vi "Main.vi"(11 "Module Admin":refnum<class "Delacor_lib_QMH_Module Admin.lvclass">) -> ()   [LabVIEW 2021, in "Signal Generator.lvlib"]
doc: "This template is based off of the Queued Message Handler design pattern and the Queued Message Handler project template that ships with LabVIEW.\n\nThe main difference is that the queue is private to this module and communication between modules is performed via Broadcast and Request events.\n\nRequest events are wrapped in public API methods and are handled in the Event Handling Loop (EHL) of this VI. Any module can register for Broadcast events sent by this module. The EHL generates messages based on user interface actions.\n\nThe Message Handling Loop (MHL) processes messages generated by the EHL, or by other messages. The messages are string values, so new messages can be added easily to the Message Cases case structure in the MHL. Each message cluster can also provide an optional value for Message Data, which is a variant that can be converted to whatever message-specific data is required.\n_____\nBased on DQMH Project Template 7.0.1.1316."
uses:
  Signal Generator.lvlib
  <vilib>/Delacor/Delacor QMH/Libraries/Module Admin_class/Delacor_lib_QMH_Module Admin.lvclass
  Module Data--cluster.ctl
  Update Parameters Argument--cluster.ctl
  <vilib>/Delacor/Delacor QMH/Libraries/Message Queue_class/Delacor_lib_QMH_Message Queue.lvclass/Delacor_lib_QMH_Message Queue.ctl
  Stop Argument--cluster.ctl
  <vilib>/Delacor/Delacor QMH/Libraries/Module Admin_class/Delacor_lib_QMH_Module Admin.lvclass/Delacor_lib_QMH_Module Admin.ctl
  Get Modules Name Argument--cluster.ctl
  Get Modules Name (Reply Payload)--cluster.ctl
  Update Parameters 2 Argument--cluster.ctl
  <vilib>/Utility/miscctls.llb/LVPointTypeDef.ctl
  <vilib>/Delacor/Delacor QMH/Libraries/Message Queue_class/Delacor_lib_QMH_Enqueue Message (Single).vi
  <vilib>/Delacor/Delacor QMH/Libraries/Module Admin_class/Delacor_lib_QMH_Get External Launch.vi
  <vilib>/Delacor/Delacor QMH/Libraries/Message Queue_class/Delacor_lib_QMH_Message Queue.lvclass
  <vilib>/measure/NI_MABase.lvlib
panel:
  out "error out":errorcluster
  out "Status":string
  in  "Simulate MHL Error":bool
  in  "Simulate EHL Error":bool
  # "Other processes communicate with this Module via its Public API (wrappers for its Request Events).\n\nThis Module communicates with other processes via its Broadcast Events.\nAny process that wants to receive these messages can register for this module's Broadcast events."
  # "This template is for the DQMH framework. See the block diagram for more information on how to use this template."
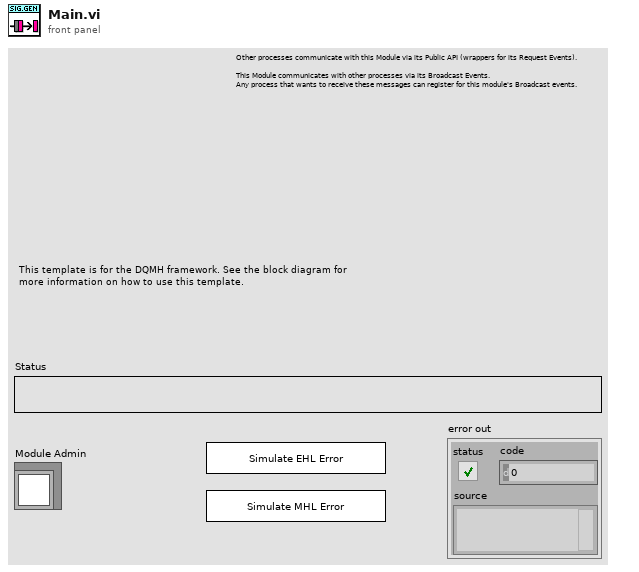
[diagram p1: front panel]
types:
  T1 = typedef "Signal Generator.lvlib/Request Events--cluster.ctl" = cluster{"Stop Module":refnum<user-event>, "Show Panel":refnum<user-event>, "Hide Panel":refnum<user-event>, "Get Module Execution Status":refnum<user-event>, "Show Diagram":refnum<user-event>, "Update Parameters":refnum<user-event>, "Private":cluster{"Start Signal Generation Loop":refnum<user-event>}, "Get Modules Name":refnum<user-event>, "Update Parameters 2":refnum<user-event>}
  T2 = typedef "Signal Generator.lvlib/Update Parameters Argument--cluster.ctl" = cluster{"amplitude":dbl, "frequency":dbl, "signal type":enum16{"Sine Wave", "Triangle Wave", "Square Wave", "Sawtooth Wave"}}
  T3 = typedef "Signal Generator.lvlib/Module Data--cluster.ctl" = cluster{"Status":string}
  T4 = enum32{"invalid lock state", "Not Locked", "Locked (No Password)", "Password-protected"}
  T5 = typedef "Signal Generator.lvlib/Stop Argument--cluster.ctl" = cluster{"Origin":string, "Exit via Stop Module Req?":bool, "Wait for Module to stop?":bool}
  T6 = typedef "Signal Generator.lvlib/Get Modules Name Argument--cluster.ctl" = cluster{"Wait Notifier":refnum<notifier>, "wait for reply":bool}
  T7 = typedef "Signal Generator.lvlib/Update Parameters 2 Argument--cluster.ctl" = cluster{"amplitude":dbl, "frequency":dbl, "signal type":enum16{"Sine Wave", "Triangle Wave", "Square Wave", "Sawtooth Wave"}}
  T8 = typedef "LVPointTypeDef.ctl" = cluster{"Horizontal":i16, "Vertical":i16}
  T9 = enum32{"Invalid", "Standard", "Closed", "Hidden", "Minimized", "Maximized"}
  T10 = typedef "Signal Generator.lvlib/Get Modules Name (Reply Payload)--cluster.ctl" = cluster{"Module Name":string, "error":errorcluster}
  T11 = enum16{"Sine Wave", "Triangle Wave", "Square Wave", "Sawtooth Wave"}
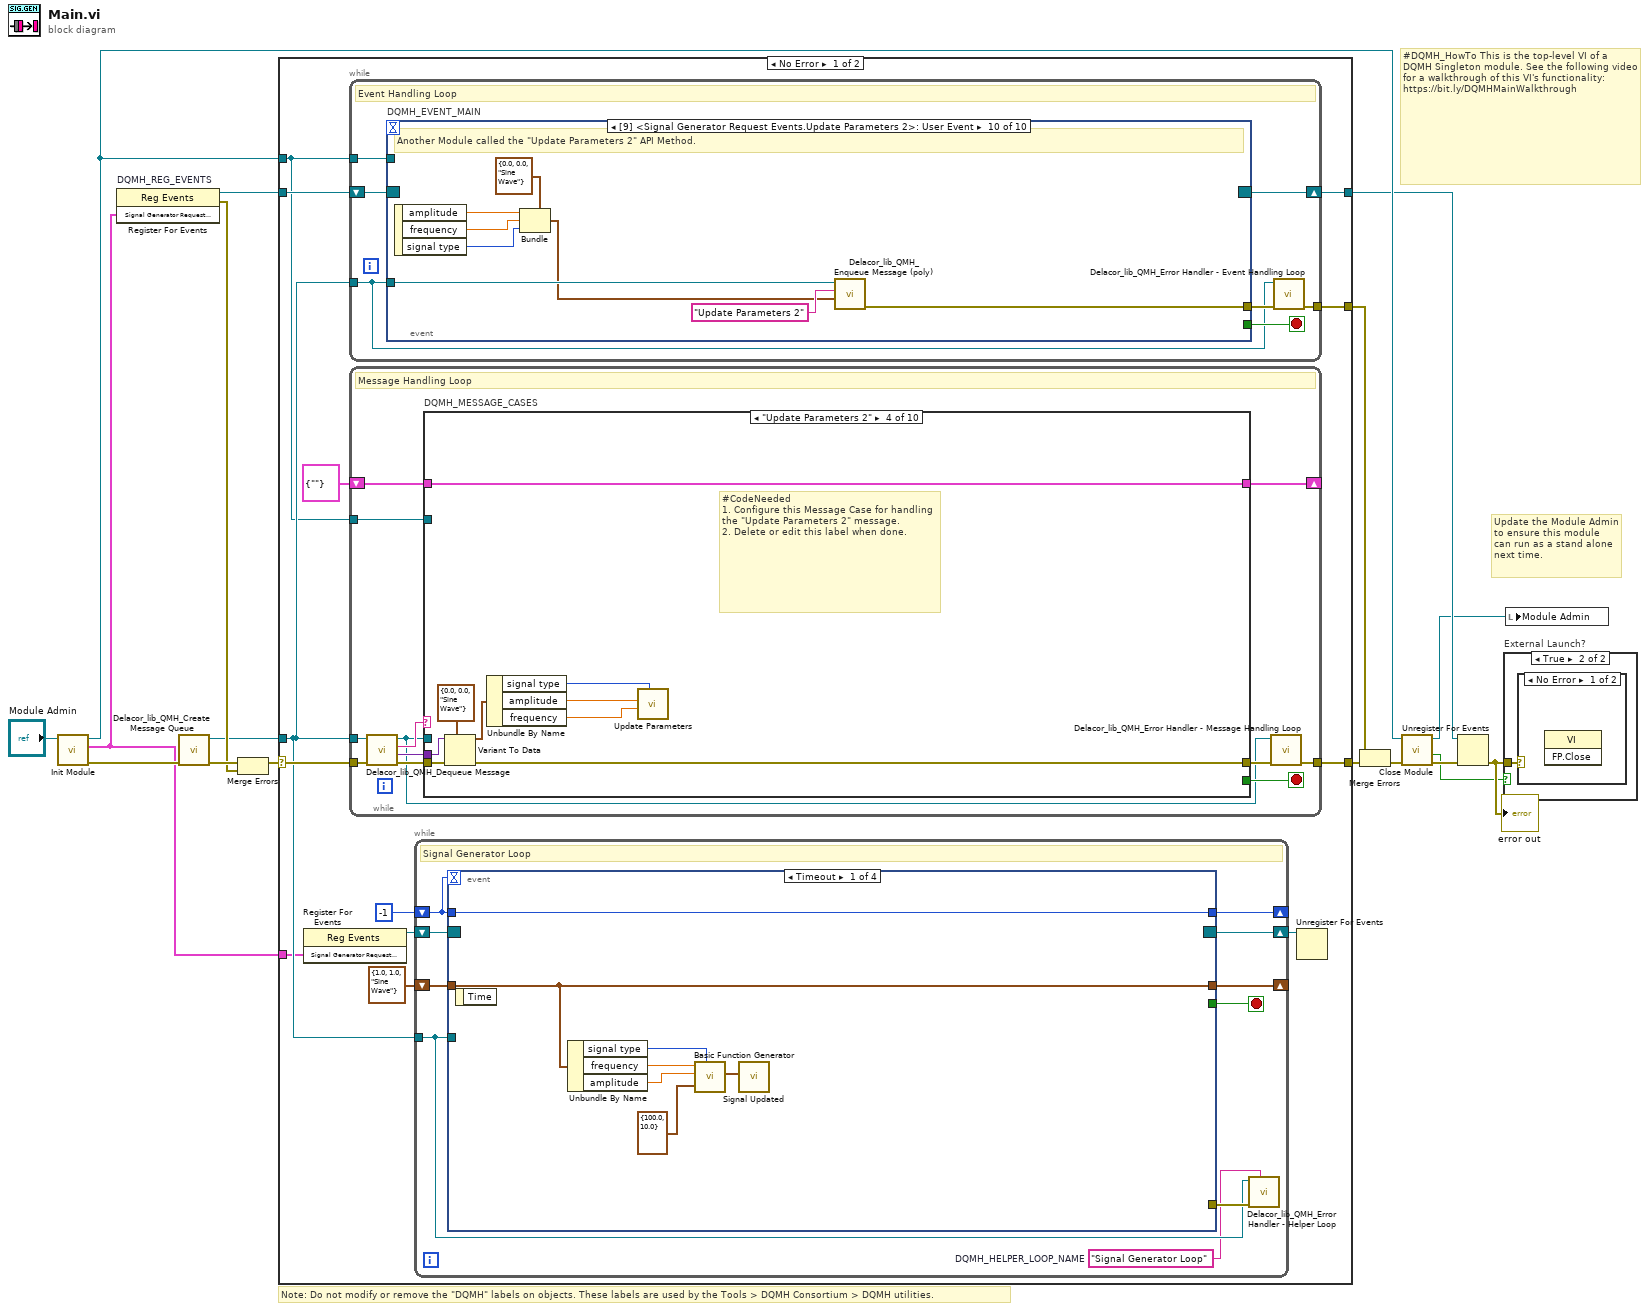
[diagram p0: block diagram]
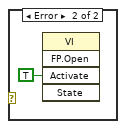
[diagram p3: hidden frame]
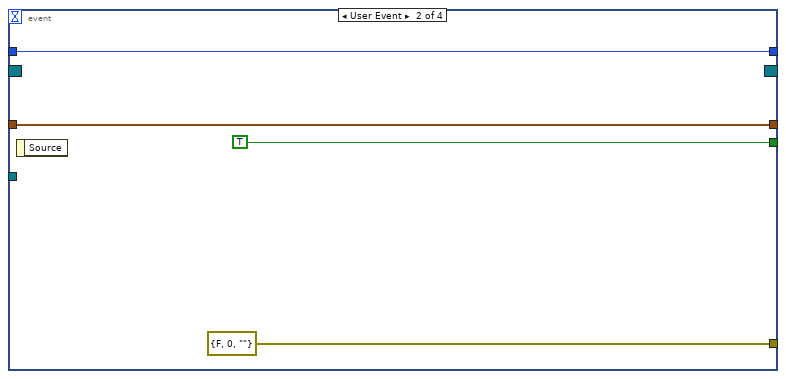
[diagram p4: hidden frame]
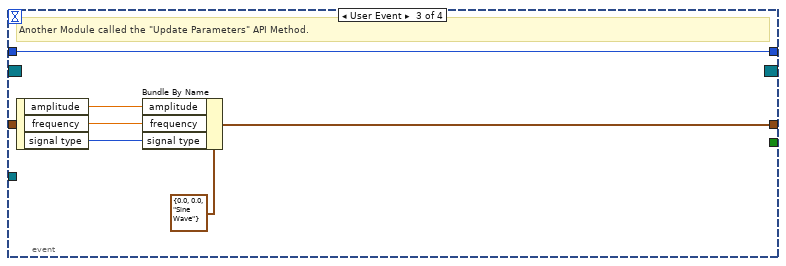
[diagram p5: hidden frame]
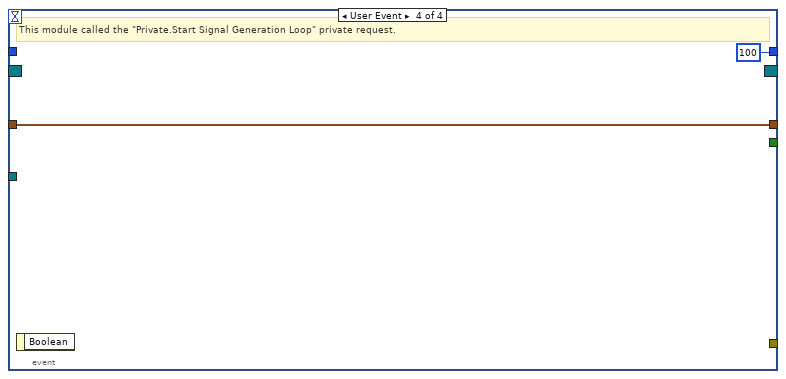
[diagram p6: hidden frame]
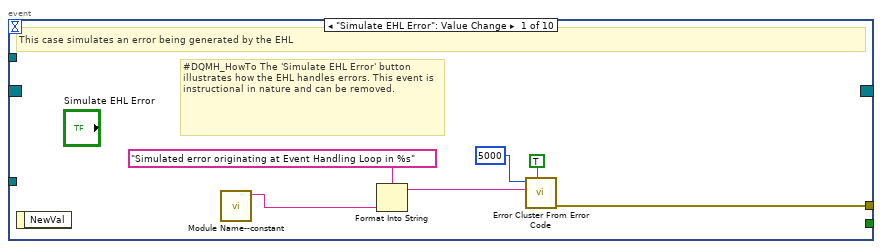
[diagram p7: hidden frame]
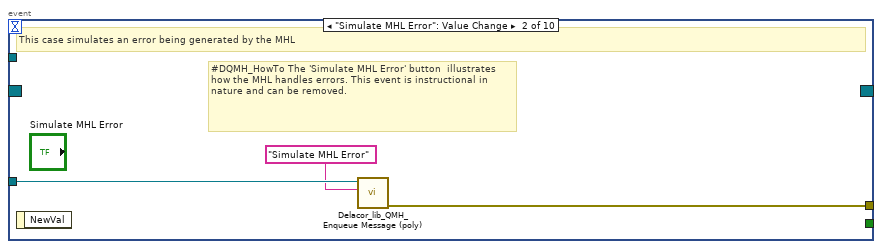
[diagram p8: hidden frame]
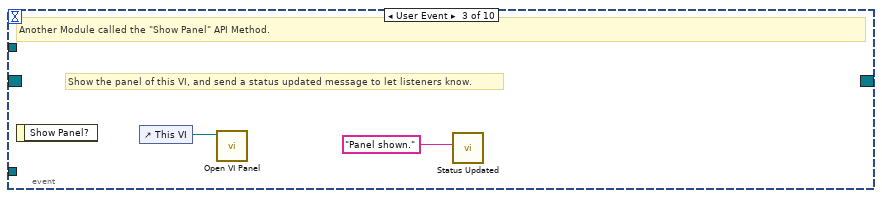
[diagram p9: hidden frame]
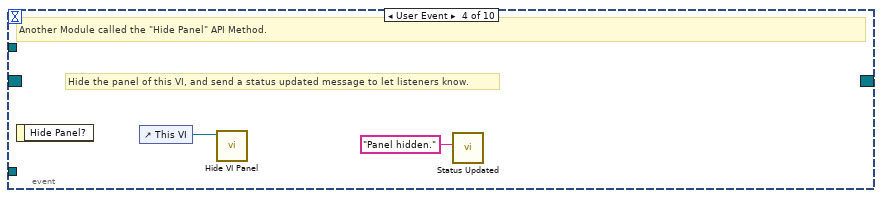
[diagram p10: hidden frame]
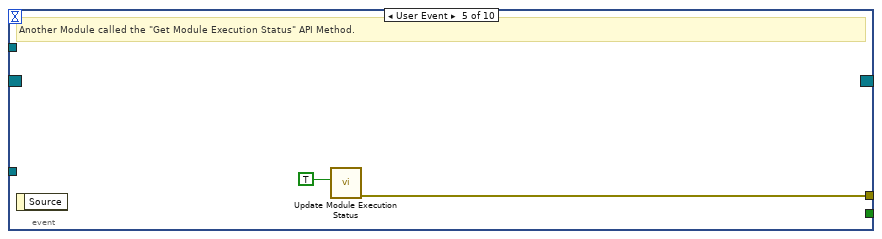
[diagram p11: hidden frame]
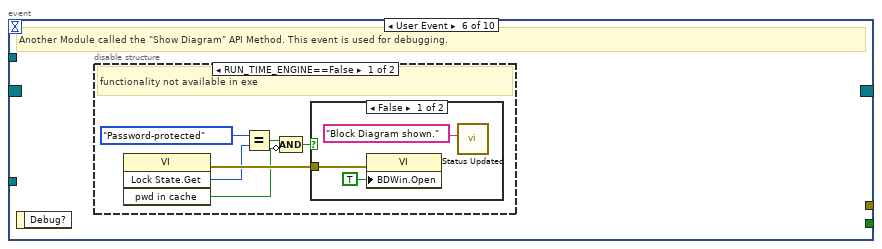
[diagram p12: hidden frame]
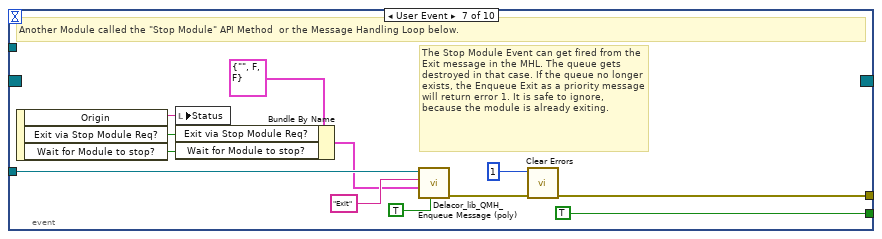
[diagram p15: hidden frame]
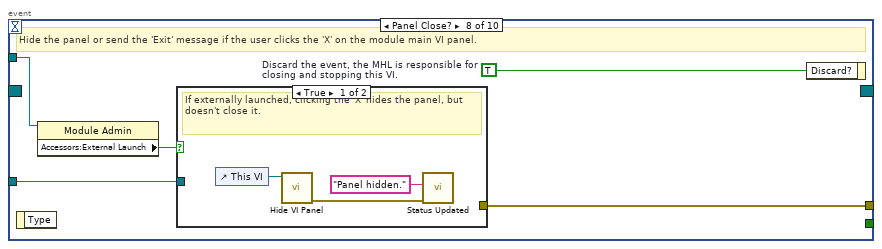
[diagram p16: hidden frame]
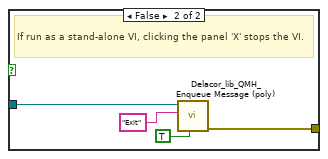
[diagram p17: hidden frame]
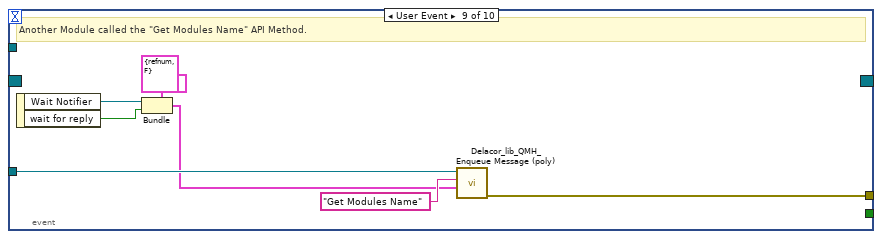
[diagram p18: hidden frame]
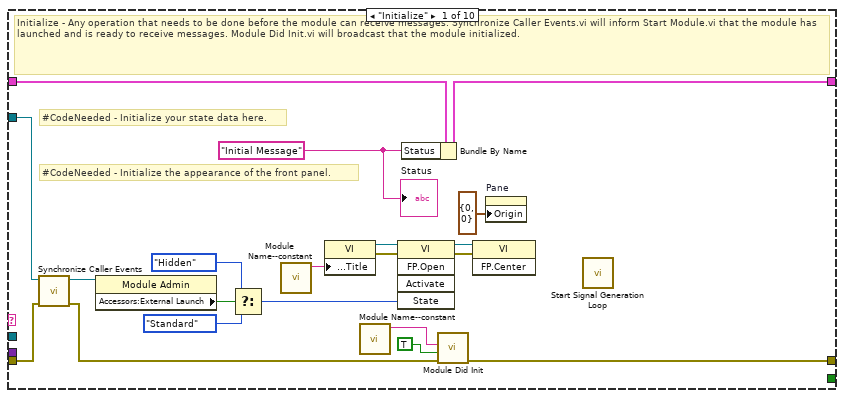
[diagram p19: hidden frame]
diagram:
  # "#DQMH_HowTo This is the top-level VI of a DQMH Singleton module. See the following video for a walkthrough of this VI's functionality: https://bit.ly/DQMHMainWalkthrough"
  # "Note: Do not modify or remove the \"DQMH\" labels on objects. These labels are used by the Tools > DQMH Consortium > DQMH utilities."
  # "Update the Module Admin to ensure this module can run as a stand alone next time."
  n1 = call "Init Module.vi"("Singleton Module Admin in"="Module Admin") -> ("error out"=w16:errorcluster, "Signal Generator Request Events"=w1:T1, "Singleton Module Admin out"=w8:refnum<class "Delacor_lib_QMH_Module Admin.lvclass">)  [unwired: 8 in]
  n2 = register-events "DQMH_REG_EVENTS"(w1) -> (reference out=w6:refnum<event-registration>, error out=w9:errorcluster)  [unwired: 2 in]
  n3 = call <vilib>:"Delacor_lib_QMH_Create Message Queue.vi"("error in"=w16) -> ("error out"=w11:errorcluster, "Message Queue"=w5:refnum<class "Delacor_lib_QMH_Message Queue.lvclass">)  [unwired: 9 in]
  n4 = Merge Errors(w11, w9) -> (w10:errorcluster)
  n5 = case shown="No Error" w10 {
    selector: w10 -> [w28 w250]
    tunnel: [w30 w249] -> w17
    tunnel: [w27 w248] -> w7
    tunnel: w6 -> [w25 w248]
    tunnel: w5 -> [w24 w243]
    tunnel: [w29 _] -> w14
    tunnel: w8 -> [w23 w244]
    tunnel: w1 -> [w22 _]
    frame No Error {
      n6 = register-events ("DQMH_HELPER_REGFOREVENTS")(w22) -> (reference out=w20:refnum<event-registration>)  [unwired: 2 in, 1 out]
      n7 = while {
        tunnel: w24 -> [w60]
        shift-right: [w63] -> w27
        shift-left: w25 -> [w64]
        tunnel: [w65] -> w29
        tunnel: w23 -> [w61]
        stop <- w62 stop-if-true
        # "Event Handling Loop"
        n8 = event "DQMH_EVENT_MAIN" shown="[9] <Signal Generator Request Events.Update Parameters 2>: User Event" {
          selector: w64 -> [_ _ _ _ _ _ _ _ _ _]
          dyn-events: [_ _ _ _ _ _ _ _ _ _] -> w63
          timeout: _ -> [_ _ _ _ _ _ _ _ _ _]
          tunnel: [_ _ _ _ _ _ TRUE ("Discard?") _ _ _] -> w62
          tunnel: w60 -> [_ w74 _ _ _ _ w98 w105 w121 w129]
          tunnel: [w72 w75 _ _ w81 _ w101 w107 w115 w122] -> w66
          tunnel: w61 -> [_ _ _ _ _ _ _ w104 _ _]
          event "Simulate EHL Error": Value Change {
            # "#DQMH_HowTo The 'Simulate EHL Error' button  illustrates how the EHL handles errors. This event is instructional in nature and can be removed."
            # "This case simulates an error being generated by the EHL"
            n9 = event-data() -> ()  [unwired: 1 in, 1 out]
            n10 = call "Module Name--constant.vi"() -> ("Module Name"=w69:string)  [unwired: 11 in]
            n11 = Format Into String(format string="Simulated error originating at Event Handling Loop in %s", w69) -> (resulting string=w70:string)  [unwired: 2 in, 1 out]
            n12 = call <vilib>:"Error Cluster From Error Code.vi"("show call chain? (False)"=TRUE, "error message (\"\")"=w70, "error code (0)"=5000) -> ("error out"=w72:errorcluster)  [unwired: 6 in]
          }
          event "Simulate MHL Error": Value Change {
            # "#DQMH_HowTo The 'Simulate MHL Error' button  illustrates how the MHL handles errors. This event is instructional in nature and can be removed."
            # "This case simulates an error being generated by the MHL"
            n13 = event-data() -> ()  [unwired: 1 in, 1 out]
            n14 = call-poly <vilib>:"Delacor_lib_QMH_Enqueue Message (poly).vi"("Message"="Simulate MHL Error", "Message Queue in"=w74) -> ("error out"=w75:errorcluster)  [unwired: 8 in, 1 out]
          }
          event User Event {
            # "Show the panel of this VI, and send a status updated message to let listeners know."
            # "Another Module called the \"Show Panel\" API Method."
            n15 = event-data() -> ()  [unwired: 1 in, 1 out]
            n16 = control-ref of="This VI"() -> (w77:refnum<vi>)
            n17 = call "Open VI Panel.vi"("VI"=w77) -> ()  [unwired: 10 in, 1 out]
            n18 = call "Status Updated.vi"("Status"="Panel shown." ("format string")) -> ()  [unwired: 10 in, 1 out]
          }
          event User Event {
            # "Hide the panel of this VI, and send a status updated message to let listeners know."
            # "Another Module called the \"Hide Panel\" API Method."
            n19 = event-data() -> ()  [unwired: 1 in, 1 out]
            n20 = control-ref of="This VI"() -> (w79:refnum<vi>)
            n21 = call "Hide VI Panel.vi"("VI"=w79) -> ()  [unwired: 10 in, 1 out]
            n22 = call "Status Updated.vi"("Status"="Panel hidden." ("format string")) -> ()  [unwired: 10 in, 1 out]
          }
          event User Event {
            # "Another Module called the \"Get Module Execution Status\" API Method."
            n23 = event-data() -> ()  [unwired: 1 in, 1 out]
            n24 = call "Update Module Execution Status.vi"("Running?"=TRUE) -> ("error out"=w81:errorcluster)  [unwired: 10 in]
          }
          event User Event {
            # "Another Module called the \"Show Diagram\" API Method. This event is used for debugging."
            n25 = event-data() -> ()  [unwired: 1 in, 1 out]
            n26 = disable-structure shown="RUN_TIME_ENGINE==False" {
              frame condition #0 (active) {
                # "functionality not available in exe"
                n27 = invoke on="Invoke Node" class="VI" method="Lock State.Get"() -> (error out=w87:errorcluster, "Get Lock State"=w86:T4, "pwd in cache"=w83:bool)  [unwired: 4 in, 1 out]
                n28 = Equal?(x=T4."Password-protected", y=w86) -> (x = y?=w84:bool)
                n29 = Compound Arithmetic op=AND(w84, invert w83) -> (w82:bool)
                n30 = case shown="False" w82 {
                  tunnel: w87 -> [w90 _]
                  frame False {
                    n31 = property on="Property Node" class="VI"(error in=w90, "BDWin.Open"=TRUE ("Block Diagram Window:Open")) -> ()  [unwired: 1 in, 2 out]
                    n32 = call "Status Updated.vi"("Status"="Block Diagram shown." ("format string")) -> ()  [unwired: 10 in, 1 out]
                  }
                  frame True {
                    # "Password-protected VI, and the password is not in the cache. Do not show the diagram."
                  }
                }
              }
              frame condition #1 {
              }
            }
          }
          event User Event {
            # "The Stop Module Event can get fired from the Exit message in the MHL. The queue gets destroyed in that case. If the queue no longer exists, the Enqueue Exit as a priority message will return error 1. It is safe to ignore, because the module is already exiting."
            # "Another Module called the \"Stop Module\" API Method  or the Message Handling Loop below."
            n33 = event-data() -> ("Origin"=w97:string, "Exit via Stop Module Req?"=w93:bool, "Wait for Module to stop?"=w92:bool)  [unwired: 1 in]
            n34 = local write "Status"(w97) -> ()
            n35 = Bundle By Name(cluster=T5 {"Origin"="", "Exit via Stop Module Req?"=FALSE, "Wait for Module to stop?"=FALSE} ("Stop Argument"), "Exit via Stop Module Req?"=w93, "Wait for Module to stop?"=w92) -> (w91:T5)
            n36 = call-poly <vilib>:"Delacor_lib_QMH_Enqueue Message (poly).vi"("Priority Message? (F)"=TRUE, "Message Data"=w91, "Message"="Exit", "Message Queue in"=w98) -> ("error out"=w102:errorcluster)  [unwired: 6 in, 1 out]
            n37 = call <vilib>:"Clear Errors.vi"("error in (no error)"=w102, "specific error code to clear (0: all)"=1) -> ("error out"=w101:errorcluster)  [unwired: 4 in, 1 out]
          }
          event Panel Close? {
            w106 = TRUE  # Discard the event, the MHL is responsible for closing and stopping this VI.
            # "Hide the panel or send the 'Exit' message if the user clicks the 'X' on the module main VI panel."
            n38 = event-data() -> ()  [unwired: 1 in, 1 out]
            n39 = property on="Property Node" class="Module Admin"(reference=w104) -> ("Accessors:External Launch"=w103:bool)  [unwired: 1 in, 2 out]
            n40 = case shown="True" w103 {
              tunnel: w105 -> [_ w113]
              tunnel: [_ w114] -> w107
              frame True {
                # "If externally launched, clicking the 'X' hides the panel, but doesn't close it."
                n41 = control-ref of="This VI"() -> (w110:refnum<vi>)
                n42 = call "Hide VI Panel.vi"("VI"=w110) -> ("error out"=w108:errorcluster)  [unwired: 10 in]
                n43 = call "Status Updated.vi"("error in"=w108, "Status"="Panel hidden." ("format string")) -> ()  [unwired: 9 in, 1 out]
              }
              frame False {
                # "If run as a stand-alone VI, clicking the panel 'X' stops the VI."
                n44 = call-poly <vilib>:"Delacor_lib_QMH_Enqueue Message (poly).vi"("Priority Message? (F)"=TRUE, "Message"="Exit", "Message Queue in"=w113) -> ("error out"=w114:errorcluster)  [unwired: 7 in, 1 out]
              }
            }
            n45 = event-data ("Event Filter Node")("Discard?"=w106) -> ()  [unwired: 1 in, 1 out]
          }
          event User Event {
            # "Another Module called the \"Get Modules Name\" API Method."
            n46 = event-data() -> ("Wait Notifier"=w117:refnum<notifier>, "wait for reply"=w116:bool)  [unwired: 1 in]
            n47 = Bundle(cluster=T6 {"Wait Notifier"=refnum, "wait for reply"=FALSE} ("Get Modules Name Argument"), "Wait Notifier"=w117, "wait for reply"=w116) -> (w118:T6)
            n48 = call-poly <vilib>:"Delacor_lib_QMH_Enqueue Message (poly).vi"("Message Data"=w118, "Message"="Get Modules Name", "Message Queue in"=w121) -> ("error out"=w115:errorcluster)  [unwired: 7 in, 1 out]
          }
          event User Event {
            # "Another Module called the \"Update Parameters 2\" API Method."
            n49 = event-data() -> ("amplitude"=w125:dbl, "frequency"=w124:dbl, "signal type"=w123:T11)  [unwired: 1 in]
            n50 = Bundle(cluster=T7 {"amplitude"=0.0, "frequency"=0.0, "signal type"=enum."Sine Wave"} ("Update Parameters 2 Argument"), "amplitude"=w125, "frequency"=w124, "signal type"=w123) -> (w126:T7)
            n51 = call-poly <vilib>:"Delacor_lib_QMH_Enqueue Message (poly).vi"("Message Data"=w126, "Message"="Update Parameters 2", "Message Queue in"=w129) -> ("error out"=w122:errorcluster)  [unwired: 7 in, 1 out]
          }
        }
        n52 = call-dynamic "Delacor_lib_QMH_Error Handler - Event Handling Loop.vi"("error in"=w66, "Message Queue in"=w60) -> ("dup error in"=w65:errorcluster)  [unwired: 8 in, 1 out]
      }
      n53 = while {
        tunnel: w24 -> [w130]
        shift-right: [w138] -> _
        shift-left: T3 {"Status"=""} ("Data Cluster") -> [w139]
        tunnel: w28 -> [w141]
        tunnel: [w133] -> w30
        tunnel: w23 -> [w134]
        stop <- w137 stop-if-true
        # "Message Handling Loop"
        n54 = call-dynamic "Delacor_lib_QMH_Dequeue Message.vi"("error in"=w141, "Message Queue in"=w130) -> ("error out"=w140:errorcluster, "Message Data"=w135:variant, "Message"=w136:string, "Message Queue out"=w131:refnum<class "Delacor_lib_QMH_Message Queue.lvclass">)  [unwired: 6 in]
        n55 = case "DQMH_MESSAGE_CASES" shown="\"Update Parameters 2\"" w136 {
          selector: w136 -> [_ _ _ _ _ _ _ _ _ w238]
          tunnel: w131 -> [_ _ _ _ _ _ _ w204 w226 _]
          tunnel: w140 -> [w159 w163 w175 w186 w189 w191 w200 w211 w232 w241]
          tunnel: [w157 w163 w165 w184 w188 w191 w199 w207 w227 w242] -> w132
          tunnel: w139 -> [w148 w162 w174 w185 w187 w190 w197 w206 w225 w239]
          tunnel: [w147 w162 w174 w185 w187 w190 w197 w206 w225 w239] -> w138
          tunnel: [_ _ _ _ _ _ _ _ w224 _] -> w137
          tunnel: w135 -> [_ _ w172 w183 _ _ _ w205 w223 _]
          tunnel: w134 -> [w149 _ _ _ _ _ _ w203 w218 _]
          frame "Initialize" {
            w143 = "Initial Message" ("Initial Message")
            # "#CodeNeeded - Initialize the appearance of the front panel."
            # "#CodeNeeded - Initialize your state data here."
            # "Initialize - Any operation that needs to be done before the module can receive messages. Synchronize Caller Events.vi will inform Start Module.vi that the module has launched and is ready to receive messages. Module Did Init.vi will broadcast that the module initialized."
            n56 = call "Synchronize Caller Events.vi"("error in"=w159, "Singleton Module Admin in"=w149) -> ("error out"=w158:errorcluster, "Singleton Module Admin out"=w144:refnum<class "Delacor_lib_QMH_Module Admin.lvclass">)  [unwired: 8 in]
            n57 = property on="Property Node" class="Module Admin"(reference=w144) -> ("Accessors:External Launch"=w153:bool)  [unwired: 1 in, 2 out]
            n58 = Select(t=T9."Hidden" ("State"), s=w153, f=T9."Standard" ("State")) -> (s? t:f=w150:T9)
            n59 = call "Module Name--constant.vi"() -> ("Module Name"=w156:string)  [unwired: 11 in]
            n60 = property on="Property Node" class="VI"("Front Panel.Title"=w156) -> (reference out=w155:refnum<vi>, error out=w161:errorcluster)  [unwired: 2 in]
            n61 = call "Module Name--constant.vi"() -> ("Module Name"=w145:string)  [unwired: 11 in]
            n62 = invoke on="Invoke Node" class="VI" method="FP.Open"(reference=w155, error in=w161, "State"=w150) -> (reference out=w154:refnum<vi>, error out=w160:errorcluster)  [unwired: 2 in, 3 out]
            n63 = Bundle By Name(cluster=w148, "Status"=w143) -> (w147:T3)
            n64 = call "Module Did Init.vi"("error in"=w158, "Initialized?"=TRUE, "Origin"=w145) -> ("error out"=w157:errorcluster)  [unwired: 8 in]
            n65 = invoke on="Invoke Node" class="VI" method="FP.Center"(reference=w154, error in=w160) -> ()  [unwired: 1 in, 3 out]
            n66 = property on="Pane" class="Pane"("Origin"=T8 {"Horizontal"=0, "Vertical"=0}) -> ()  [unwired: 2 in, 2 out]
            n67 = call "Start Signal Generation Loop.vi"() -> ()  [unwired: 11 in, 1 out]
            "Status" <- w143
          }
          frame "---Module Specific---" {
            # "Separator -- The following cases handle messages specific to this Module."
          }
          frame "Get Modules Name" {
            n68 = Variant To Data(error in=w175, type=T6 {"Wait Notifier"=refnum, "wait for reply"=FALSE} ("Get Modules Name Argument"), Variant=w172) -> (data=w170:T6, error out=w173:errorcluster)
            n69 = Unbundle By Name(w170) -> ("Wait Notifier"=w169:refnum<notifier>, "wait for reply"=w168:bool)
            n70 = Bundle By Name(cluster=T10 {"Module Name"="", "error"={"status"=FALSE, "code"=0, "source"=""}} ("Get Modules Name (Reply Payload)"), "Module Name"="LV Turkey Signal Generator") -> (w167:T10)
            n71 = Merge Errors(w173) -> (w165:errorcluster)
            n72 = case "DQMH_FIRE_NOTIFIER" shown="True" w168 {
              tunnel: w169 -> [_ w177]
              tunnel: w167 -> [_ w176]
              frame False {
              }
              frame True {
                n73 = Send Notification(notification=w176, notifier=w177) -> ()  [unwired: 1 in, 2 out]
              }
            }
          }
          frame "Update Parameters 2" {
            # "#CodeNeeded\n1. Configure this Message Case for handling the \"Update Parameters 2\" message.\n2. Delete or edit this label when done."
            n74 = Variant To Data(error in=w186, type=T7 {"amplitude"=0.0, "frequency"=0.0, "signal type"=enum."Sine Wave"} ("Update Parameters 2 Argument"), Variant=w183) -> (data=w181:T7, error out=w184:errorcluster)
            n75 = Unbundle By Name(w181) -> ("signal type"=w178:T11, "amplitude"=w180:dbl, "frequency"=w179:dbl)
            n76 = call "Update Parameters.vi"("signal type"=w178, "frequency"=w179, "amplitude"=w180) -> ()  [unwired: 8 in, 1 out]
          }
          frame "---Copy This Frame---" {
            # "Duplicate this frame when creating new messages.  Change this comment in the duplicated frame to describe this message."
            n77 = Merge Errors(w189) -> (w188:errorcluster)
          }
          frame "---Exit and Error Handling---" {
            # "Separator - The following cases handle errors and exit messages."
          }
          frame "Simulate MHL Error" {
            # "#DQMH_HowTo The 'Simulate MHL Error' button  illustrates how the MHL handles errors. This event is instructional in nature and can be removed."
            # "Simulate an error occurring at the MHL"
            n78 = call "Module Name--constant.vi"() -> ("Module Name"=w193:string)  [unwired: 11 in]
            n79 = Format Into String(format string="Simulated error originating at Message Handling Loop in %s", w193) -> (resulting string=w194:string)  [unwired: 2 in, 1 out]
            n80 = call <vilib>:"Error Cluster From Error Code.vi"("show call chain? (False)"=TRUE, "error message (\"\")"=w194, "error code (0)"=5001) -> ("error out"=w198:errorcluster)  [unwired: 6 in]
            n81 = Merge Errors(w200, w198) -> (w199:errorcluster)
          }
          frame "Error" {
            # "#CodeRecommended - If the module is running in standalone mode (External Launch = FALSE), this code will pop up an error dialog and call the 'Exit' message if an error occurs. Add more fine-grained error management here."
            # "Error - Check the error message data and respond accordingly. This message is sent by the \"Error Handler\" VIs at the end of each loop in this application."
            n82 = property on="Property Node" class="Module Admin"(reference=w203) -> ("Accessors:External Launch"=w202:bool)  [unwired: 1 in, 2 out]
            n83 = Variant To Data(error in=w211, type=errorcluster {"status"=FALSE, "code"=0, "source"=""} ("error constant"), Variant=w205) -> (data=w201:errorcluster, error out=w209:errorcluster)
            n84 = local write "error out"(w201) -> ()
            n85 = call "Error Reported.vi"("Error"=w201) -> ()  [unwired: 10 in, 1 out]
            n86 = case shown="False" w202 {
              tunnel: [w216 _] -> w208
              tunnel: w204 -> [w214 _]
              tunnel: w201 -> [w215 _]
              frame False {
                n87 = disable-structure shown="Default" {
                  disable-tunnel: w215 -> [w217 _]
                  frame condition #0 (active) {
                    # "If the module is running standalone, then pop up an error dialog and call the \"Exit\" message."
                    n88 = call <vilib>:"Simple Error Handler.vi"("error in (no error)"=w217) -> ()  [unwired: 4 in, 5 out]
                  }
                  frame condition #1 {
                    # "To prevent the Simple Error Handler VI from being loaded (e.g. when deploying to a Real-Time target), add the Conditional Disable Symbol \"DQMH_Disable_SEH\" to your project and set it to TRUE."
                  }
                }
                n89 = call-poly <vilib>:"Delacor_lib_QMH_Enqueue Message (poly).vi"("Priority Message? (F)"=TRUE, "Message"="Exit", "Message Queue in"=w214) -> ("error out"=w216:errorcluster)  [unwired: 7 in, 1 out]
              }
              frame True {
                # "If the module was launched externally, calling the Error Reported broadcast VI is the only action performed by the \"Error\" message. The module's caller can then process the error appropriately."
              }
            }
            n90 = Merge Errors(w209, w208) -> (w207:errorcluster)
          }
          frame "Exit" {
            w222 = 91  # 91: not all Exit messages will have an argument
            w224 = TRUE  # Stop the VI
            # "Release the message queue reference"
            # "#CodeNeeded - Add any required cleanup code here."
            # "Exit - Exit the application."
            n91 = Variant To Data(error in=w232, type=T5 {"Origin"="", "Exit via Stop Module Req?"=FALSE, "Wait for Module to stop?"=FALSE} ("Stop Argument"), Variant=w223) -> (data=w220:T5, error out=w229:errorcluster)
            n92 = call <vilib>:"Clear Errors.vi"("error in (no error)"=w229, "specific error code to clear (0: all)"=w222) -> ("error out"=w231:errorcluster)  [unwired: 4 in, 1 out]
            n93 = control-ref of="This VI"() -> (w219:refnum<vi>)
            n94 = call-dynamic "Delacor_lib_QMH_Release Message Queue.vi"("error in"=w231, "Message Queue"=w226) -> ("error out"=w230:errorcluster)  [unwired: 9 in]
            n95 = call "Handle Exit.vi"("Stop Argument"=w220, "Admin in"=w218, "VI reference"=w219) -> ("error out"=w228:errorcluster)  [unwired: 7 in, 1 out]
            n96 = Merge Errors(w230, w228) -> (w227:errorcluster)
            n97 = call "Error Reported.vi"("Error"=w227) -> ()  [unwired: 10 in, 1 out]
          }
          frame Default {
            # "'Default' case only runs if there is a message that isn't defined in any of the other cases.  Output a programming error."
            n98 = call "Module Name--constant.vi"() -> ("Module Name"=w237:string)  [unwired: 11 in]
            n99 = Format Into String(format string="The invalid message string \"%s\" was received in the Message Handling Loop for module \"%s\".", w238, w237) -> (resulting string=w233:string)  [unwired: 2 in, 1 out]
            n100 = call <vilib>:"Error Cluster From Error Code.vi"("show call chain? (False)"=TRUE, "error message (\"\")"=w233, "error code (0)"=1) -> ("error out"=w240:errorcluster)  [unwired: 6 in]
            n101 = Merge Errors(w241, w240) -> (w242:errorcluster)
          }
        }
        n102 = call-dynamic "Delacor_lib_QMH_Error Handler - Message Handling Loop.vi"("error in"=w132, "Message Queue in"=w131) -> ("dup error in"=w133:errorcluster)  [unwired: 8 in, 1 out]
      }
      n103 = while "DQMH_HELPER_LOOP" {
        shift-right: [w40] -> _
        shift-left: -1 -> [w39]
        shift-right: [w37] -> w21
        shift-left: w20 -> [w38]
        tunnel: w24 -> [w34]
        shift-right: [w32] -> _
        shift-left: T2 {"amplitude"=1.0, "frequency"=1.0, "signal type"=enum."Sine Wave"} ("Update Parameters Argument") -> [w31]
        stop <- w36 stop-if-true
        w33 = "Signal Generator Loop"  # DQMH_HELPER_LOOP_NAME
        # "Signal Generator Loop"
        n104 = event "DQMH_HELPER_EVENT_STRUCTURE" shown="[0] Timeout" {
          selector: w38 -> [_ _ _ _]
          dyn-events: [_ _ _ _] -> w37
          timeout: w39 -> [_ _ _ _]
          tunnel: w39 -> [w47 w51 w57 _]
          tunnel: [w47 w51 w57 100] -> w40
          tunnel: [_ TRUE _ _] -> w36
          tunnel: [_ errorcluster {"status"=FALSE, "code"=0, "source"=""} ("error constant") _ _] -> w35
          tunnel: w34 -> [_ _ _ _]
          tunnel: [w46 w48 w52 w59] -> w32
          tunnel: w31 -> [w46 w48 _ w59]
          event Timeout {
            n105 = event-data() -> ()  [unwired: 1 in, 1 out]
            n106 = Unbundle By Name(w46) -> ("signal type"=w43:T11, "frequency"=w45:dbl, "amplitude"=w44:dbl)
            n107 = call <vilib>:"Basic Function Generator.vi"("sampling info"=cluster{"Fs":dbl, "#s":dbl} {"Fs"=100.0, "#s"=10.0}, "signal type"=w43, "amplitude"=w44, "frequency"=w45) -> ("signal out"=w41:waveform(dbl))  [unwired: 5 in, 2 out]
            n108 = call "Signal Updated.vi"("signal"=w41) -> ()  [unwired: 10 in, 1 out]
          }
          event User Event {
            n109 = event-data() -> ()  [unwired: 1 in, 1 out]
          }
          event User Event {
            # "Another Module called the \"Update Parameters\" API Method."
            n110 = event-data() -> ("amplitude"=w55:dbl, "frequency"=w54:dbl, "signal type"=w53:T11)  [unwired: 1 in]
            n111 = Bundle By Name(cluster=T2 {"amplitude"=0.0, "frequency"=0.0, "signal type"=enum."Sine Wave"} ("Update Parameters Argument"), "amplitude"=w55, "frequency"=w54, "signal type"=w53) -> (w52:T2)
          }
          event User Event {
            # "This module called the \"Private.Start Signal Generation Loop\" private request."
            n112 = event-data() -> ()  [unwired: 1 in, 1 out]
          }
        }
        n113 = call-dynamic "Delacor_lib_QMH_Error Handler - Helper Loop.vi"("Error Debug"=w33, "error in"=w35, "Message Queue in"=w34) -> ()  [unwired: 7 in, 2 out]
      }
      n114 = Unregister For Events(event registration refnum=w21) -> ()  [unwired: 1 in, 1 out]
    }
    frame Error {
      # "Synchronize Caller Events.vi will inform Start Module.vi that the module has launched and will let the code calling Start Module.vi register for broadcasts and would permit the caller receive the broadcast that an error occurred at launch time."
      n115 = call-dynamic "Delacor_lib_QMH_Release Message Queue.vi"("error in"=w250, "Message Queue"=w243) -> ("error out"=w249:errorcluster)  [unwired: 9 in]
      n116 = call "Synchronize Caller Events.vi"("Singleton Module Admin in"=w244) -> ("error out"=w251:errorcluster)  [unwired: 9 in, 1 out]
      n117 = call "Module Name--constant.vi"() -> ("Module Name"=w247:string)  [unwired: 11 in]
      n118 = Format Into String(format string="An error occurred during initialization. %s is no longer running.", w247) -> (resulting string=w245:string)  [unwired: 2 in, 1 out]
      n119 = Merge Errors(w249, w251) -> (w252:errorcluster)
      n120 = call "Error Reported.vi"("Additional Information"=w245, "Error"=w252) -> ()  [unwired: 9 in, 1 out]
    }
  }
  n121 = Merge Errors(w14, w17) -> (w13:errorcluster)
  n122 = call "Close Module.vi"("error in"=w13, "Module Admin in"=w8) -> ("error out"=w15:errorcluster, "External Launch"=w2:bool, "Module Admin out"=w3:refnum<class "Delacor_lib_QMH_Module Admin.lvclass">)  [unwired: 7 in]
  n123 = Unregister For Events(event registration refnum=w7, error in=w15) -> (error out=w12:errorcluster)
  "error out" <- w12
  n124 = case "External Launch?" shown="True" w2 {
    tunnel: w12 -> [_ w253]
    frame False {
    }
    frame True {
      n125 = case shown="No Error" w253 {
        frame No Error {
          n126 = invoke on="Invoke Node" class="VI" method="FP.Close"() -> ()  [unwired: 3 in, 3 out]
        }
        frame Error {
          n127 = invoke on="Invoke Node" class="VI" method="FP.Open"("Activate"=TRUE ("Activate?")) -> ()  [unwired: 4 in, 5 out]
        }
      }
    }
  }
  n128 = local write "Module Admin"(w3) -> ()
